vi "Gen_Test_Single_Cell.vi"() -> ()   [LabVIEW 2020]
uses:
  Device-Interface-Layer/Chrg_Dschrg.vi
panel:
  in  "Output Safety":T1
  in  "filepath":path
  in  "Batteryname":string
  in  "Starting Cycle":i32
  out "PS error out":errorcluster
  out "PS VIS resource name out":refnum<visa-resource-name>
  out "data task error out":errorcluster
  out "data task out":refnum<k21>
  in  "Charge Current Cutoff":dbl
  in  "Charge Current Setpoint 2":dbl format="%#.6g"
  in  "charge Voltage Setpoint  2":dbl format="%#.6g"
  in  "Wait time":dbl
  in  "Discharge Current Cutoff":dbl
  in  "Discharge Current Setpoint":dbl format="%#.6g"
  in  "Discharge Voltage Setpoint":dbl format="%#.6g"
  in  "data task error in":errorcluster
  in  "Data Task in":refnum<k21>
  in  "NHR VISA":refnum<visa-resource-name>
  in  "NHR error in":errorcluster
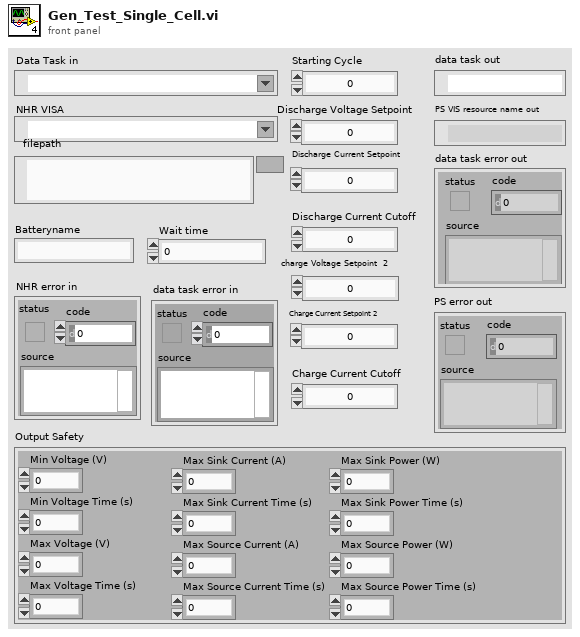
[diagram p1: front panel]
types:
  T1 = cluster{"Min Voltage (V)":dbl, "Min Voltage Time (s)":dbl, "Max Voltage (V)":dbl, "Max Voltage Time (s)":dbl, "Max Sink Current (A)":dbl, "Max Sink Current Time (s)":dbl, "Max Source Current (A)":dbl, "Max Source Current Time (s)":dbl, "Max Sink Power (W)":dbl, "Max Sink Power Time (s)":dbl, "Max Source Power (W)":dbl, "Max Source Power Time (s)":dbl}
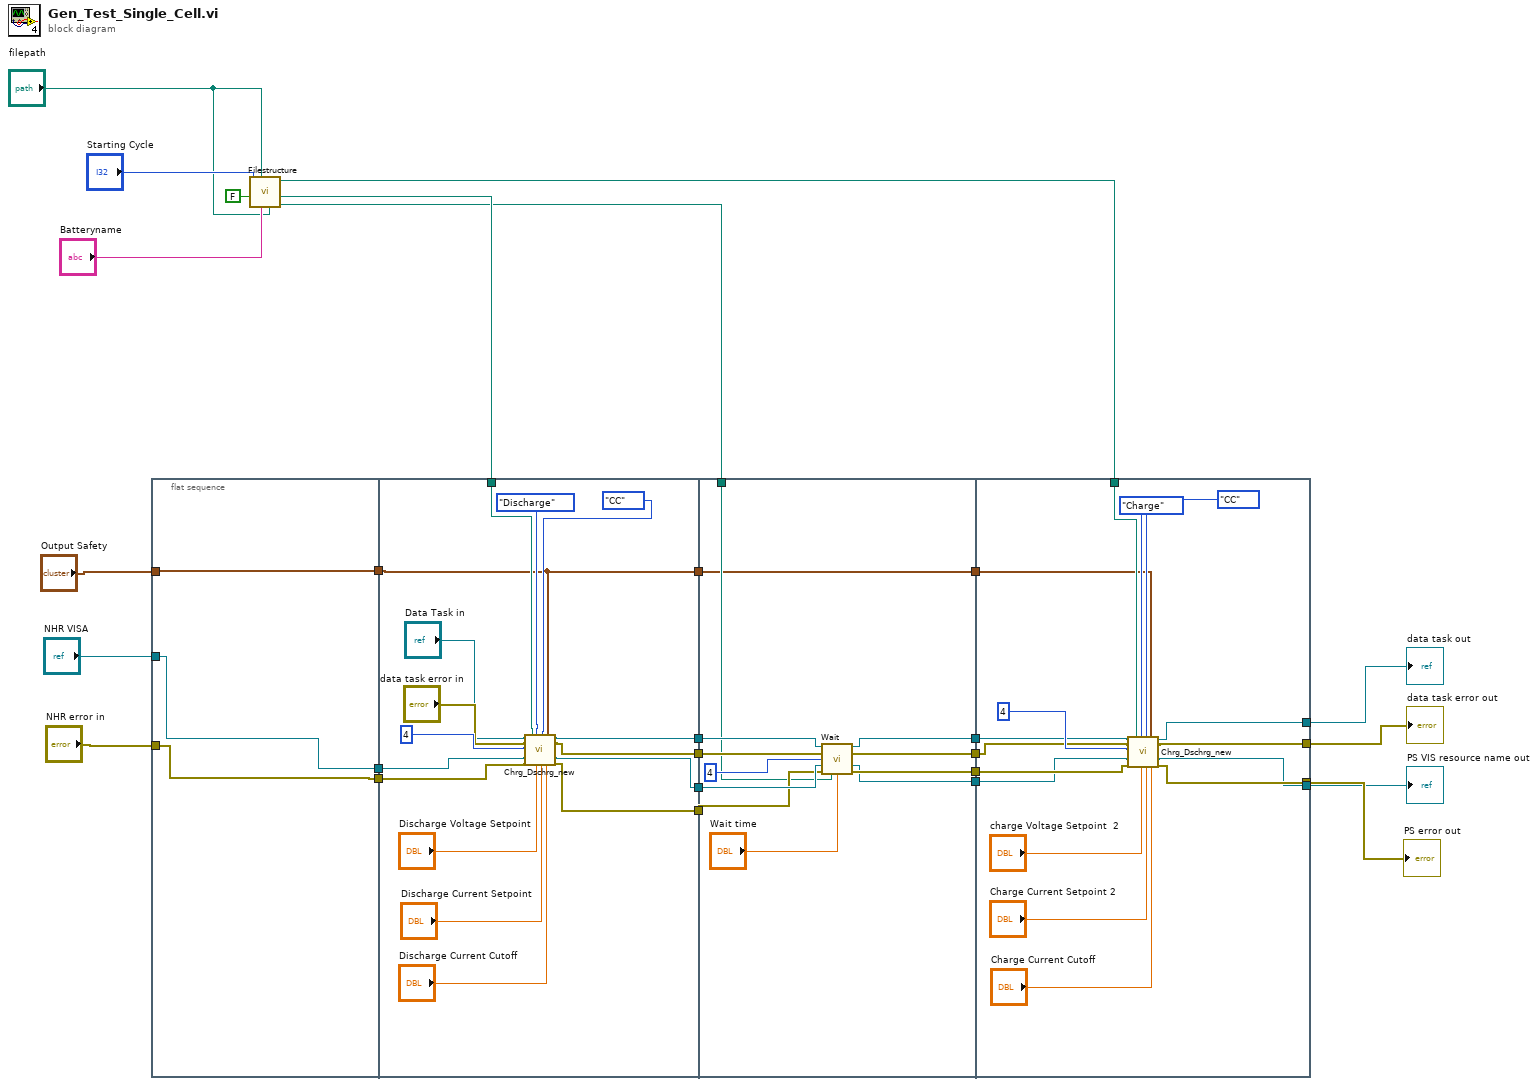
[diagram p0: block diagram]
diagram:
  n1 = flat-sequence {
    tunnel: "NHR error in" -> [w29]
    tunnel: "NHR VISA" -> [w30]
    tunnel: [w30] -> w25
    tunnel: [w29] -> w24
    tunnel: "Output Safety" -> [w28]
    tunnel: [w28] -> w4
    tunnel: w25 -> [w38]
    tunnel: w24 -> [w39]
    tunnel: [w46] -> w23
    tunnel: [w45] -> w22
    tunnel: [w44] -> w21
    tunnel: [w43] -> w20
    tunnel: w8 -> [w34]
    tunnel: w4 -> [w31]
    tunnel: [w31] -> w3
    tunnel: w23 -> [w58]
    tunnel: w22 -> [w57]
    tunnel: w21 -> [w55]
    tunnel: w20 -> [w54]
    tunnel: [w47] -> w19
    tunnel: [w52] -> w18
    tunnel: [w51] -> w17
    tunnel: [w50] -> w16
    tunnel: w7 -> [w49]
    tunnel: w3 -> [w48]
    tunnel: [w48] -> w2
    tunnel: w19 -> [w67]
    tunnel: w18 -> [w68]
    tunnel: w17 -> [w71]
    tunnel: w16 -> [w70]
    tunnel: [w62] -> w15
    tunnel: [w61] -> w14
    tunnel: [w59] -> w13
    tunnel: [w60] -> w12
    tunnel: w6 -> [w66]
    tunnel: w2 -> [w63]
    frame #0 {
    }
    frame #1 {
      n2 = call "Chrg_Dschrg_new.vi"("Data Task in"="Data Task in", "data task error in"="data task error in", "#DAQ outputs (1-13)"=4, "PS VISA in"=w38, "PS error in"=w39, "DischargeCyclePath"=w34, "Charge/discharge"=enum8{"Charge", "Discharge"}."Discharge", "Charge/Discharge Voltage Setpoint"="Discharge Voltage Setpoint", "CC or CCCV"=enum16{"CC", "CCCV"}."CC", "Current Setpoint"="Discharge Current Setpoint", "Output Safety"=w31, "Current Cutoff"="Discharge Current Cutoff") -> ("data task out"=w46:refnum<k21>, "data task error out"=w45:errorcluster, "PS VIS resource name out"=w44:refnum<visa-resource-name>, "PS error out"=w43:errorcluster)  [unwired: 4 in]
    }
    frame #2 {
      n3 = call "Wait.vi"("Data Task in"=w58, "data task error in"=w57, "#DAQ outputs (1-13)"=4, "PS VISA in"=w55, "PS error in"=w54, "Wait Filepath"=w49, "Wait time"="Wait time") -> ("data task out"=w47:refnum<k21>, "data task error out"=w52:errorcluster, "PS Visa Out"=w50:refnum<visa-resource-name>, "PS error out"=w51:errorcluster)  [unwired: 5 in]
    }
    frame #3 {
      n4 = call "Chrg_Dschrg_new.vi"("Data Task in"=w67, "data task error in"=w68, "#DAQ outputs (1-13)"=4, "PS VISA in"=w70, "PS error in"=w71, "DischargeCyclePath"=w66, "Charge/discharge"=enum8{"Charge", "Discharge"}."Charge", "Charge/Discharge Voltage Setpoint"="charge Voltage Setpoint  2", "CC or CCCV"=enum16{"CC", "CCCV"}."CC", "Current Setpoint"="Charge Current Setpoint 2", "Output Safety"=w63, "Current Cutoff"="Charge Current Cutoff") -> ("data task out"=w59:refnum<k21>, "data task error out"=w60:errorcluster, "PS VIS resource name out"=w61:refnum<visa-resource-name>, "PS error out"=w62:errorcluster)  [unwired: 4 in]
    }
  }
  n5 = call "Filestructure.vi"("Discharge filepath"="filepath", "Batteryname"="Batteryname", "Charge filepath"="filepath", "In for loop"=FALSE, "Starting Cycle"="Starting Cycle") -> ("DischargeWaitPath"=w7:path, "DischargeCyclePath"=w8:path, "ChargeCyclePath"=w6:path)  [unwired: 2 in, 2 out]
  "PS error out" <- w15
  "PS VIS resource name out" <- w14
  "data task out" <- w13
  "data task error out" <- w12
